vi "read_data_spindle_load_mt_connect (SubVI).vi"(8 "error in (no error)":errorcluster, 11 "URL":string="http://amrcadp:5000/current?&path=//") -> (0 "error out":errorcluster, 3 "number":dbl[](array[numeric]))   [LabVIEW 2017]
uses:
  <vilib>/xml/Load XML String.vi
  <vilib>/xml/Close Reference(Node).vi
  <vilib>/addons/internet/NI_InternetTK_Core_VIs.lvlib
  <vilib>/xml/NI_XML.lvlib
  <resource>/objmgr/DOMUserDefRef.rc
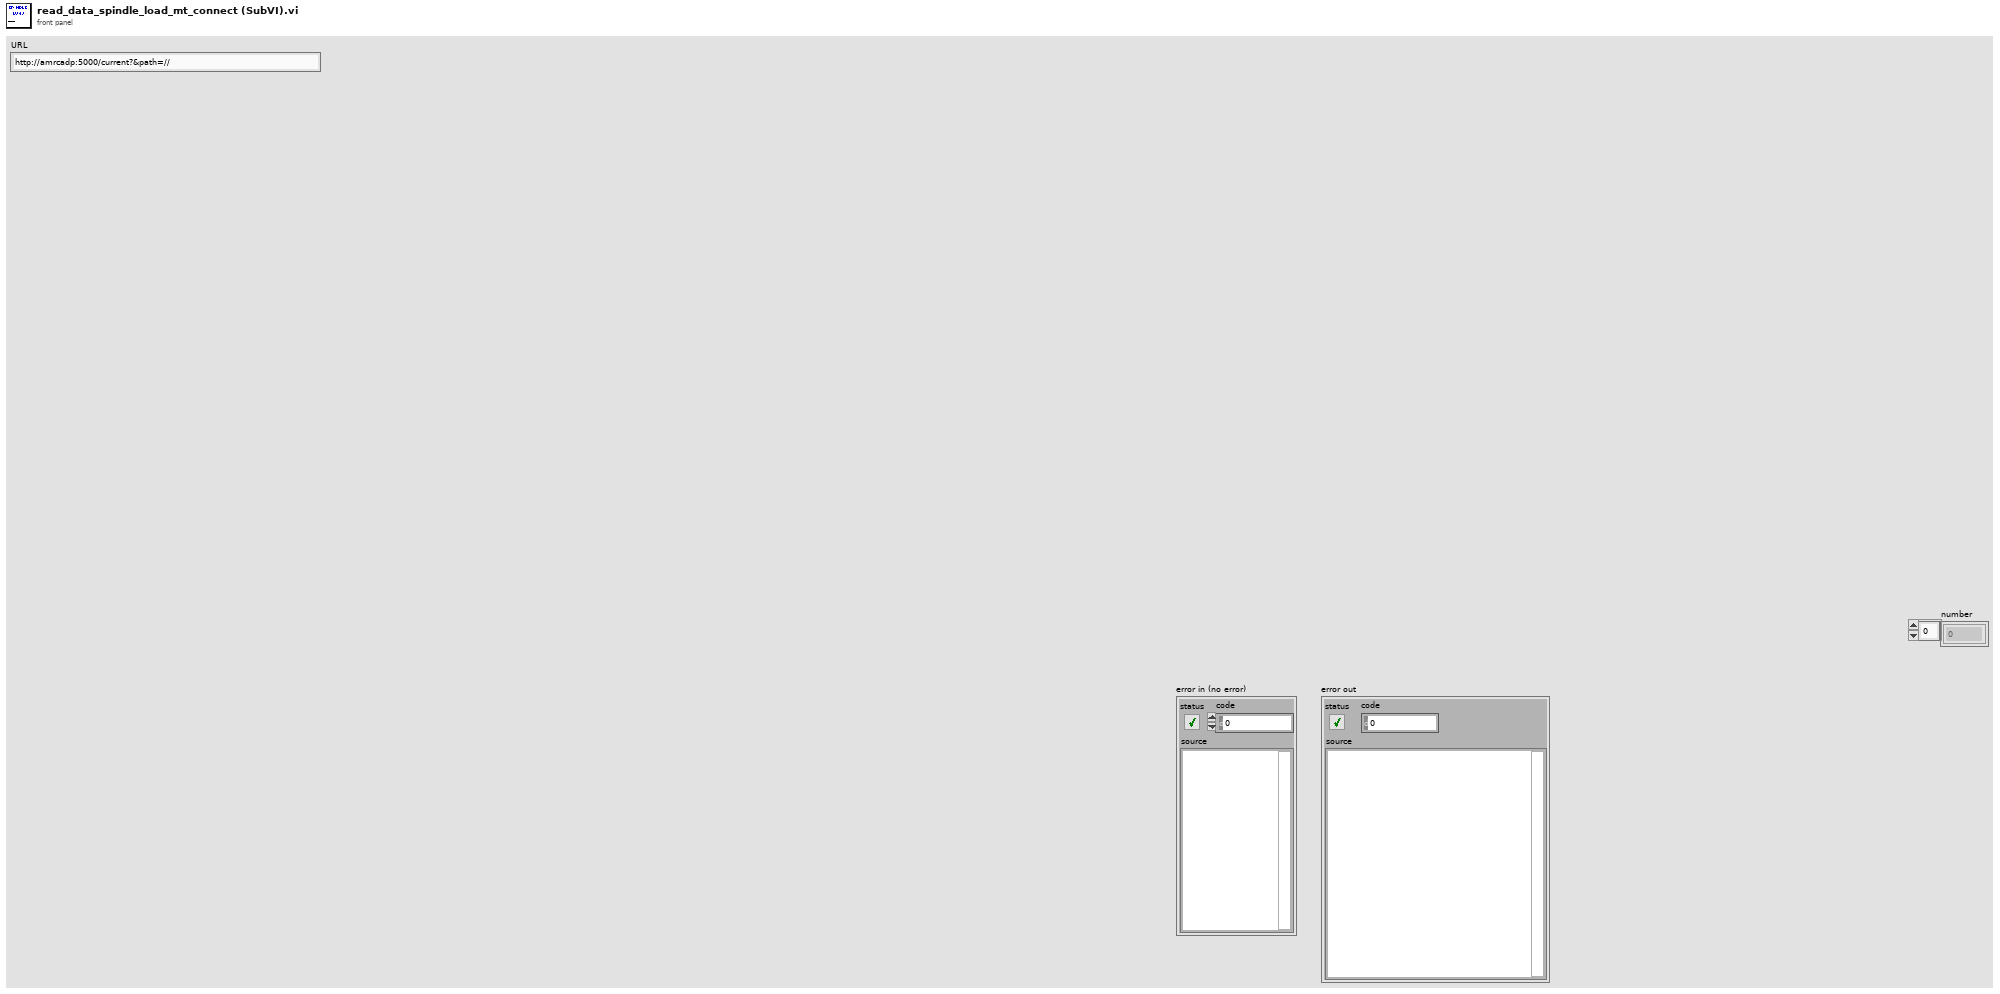
[diagram p1: front panel]
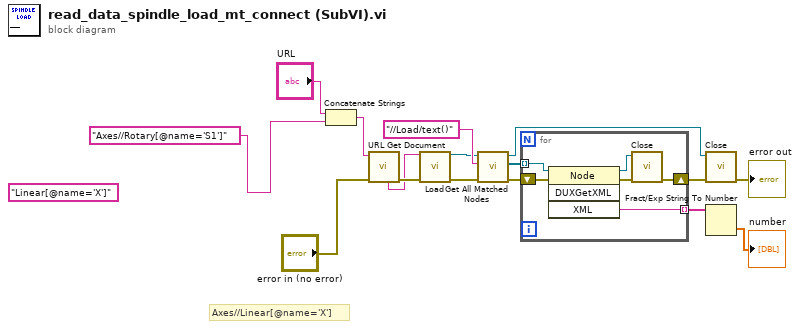
[diagram p0: block diagram]
diagram:
  (unwired) "Linear[@name='X']" ("URL")
  # "Axes//Linear[@name='X']"
  n1 = Concatenate Strings("URL", "Axes//Rotary[@name='S1']" ("URL")) -> (w3:string)
  n2 = call <vilib>:"URL Get Document.vi"("error in (no error)"="error in (no error)", "URL"=w3) -> ("error out"=w15:errorcluster, "content"=w13:string)  [unwired: 5 in, 3 out]
  n3 = call-poly <vilib>:"Load.vi"("XML string"=w13, "error in (no error)"=w15) -> ("DOM document out"=w10:refnum<k20>, "error out"=w11:errorcluster)  [unwired: 11 in, 1 out]
  n4 = call <vilib>:"Get All Matched Nodes.vi"("error in (no error)"=w11, "XPath expression"="//Load/text()", "node in"=w10) -> ("error out"=w8:errorcluster, "node result array"=w7:refnum<k20>[], "node out"=w12:refnum<k20>)  [unwired: 6 out]
  n5 = for {
    tunnel: w7 -> [w18] mode=indexing
    shift-right: [w20] -> w9
    shift-left: w8 -> [w19]
    tunnel: [w17] -> w6 mode=indexing
    n6 = invoke on="Invoke Node" class="Node" method="DUXGetXML"(reference=w18, error in=w19) -> (reference out=w21:refnum<k20>, error out=w22:errorcluster, "XML"=w17:string)  [unwired: 2 in, 1 out]
    n7 = call-poly <vilib>:"Close.vi"("error in (no error)"=w22, "node"=w21) -> ("error out"=w20:errorcluster)  [unwired: 7 out]
  }
  n8 = call-poly <vilib>:"Close.vi"("error in (no error)"=w9, "node"=w12) -> ("error out"=→"error out":errorcluster)  [unwired: 7 out]
  n9 = Fract/Exp String To Number(string=w6) -> (number=→"number":dbl[])  [unwired: 3 in, 1 out]
